vi "Acquire.vi"(8 "error in (no error)":errorcluster, 10 "Capacitive Readout Notifier":refnum<notifier>, 11 "Hardware Refs In":T1={"IP Address"="Simulator", "Handle"=0, "Refresh Time (ms)"=0.0}) -> (0 "error out":errorcluster, 3 "Hardware Refs Out":T1={"IP Address"="Simulator", "Handle"=0, "Refresh Time (ms)"=0.0})   [LabVIEW 2013, in "Capacitive.lvlib"]
uses:
  Capacitive.lvlib
  Hardware Configuration.ctl
  Capacitive Signal Cluster.ctl
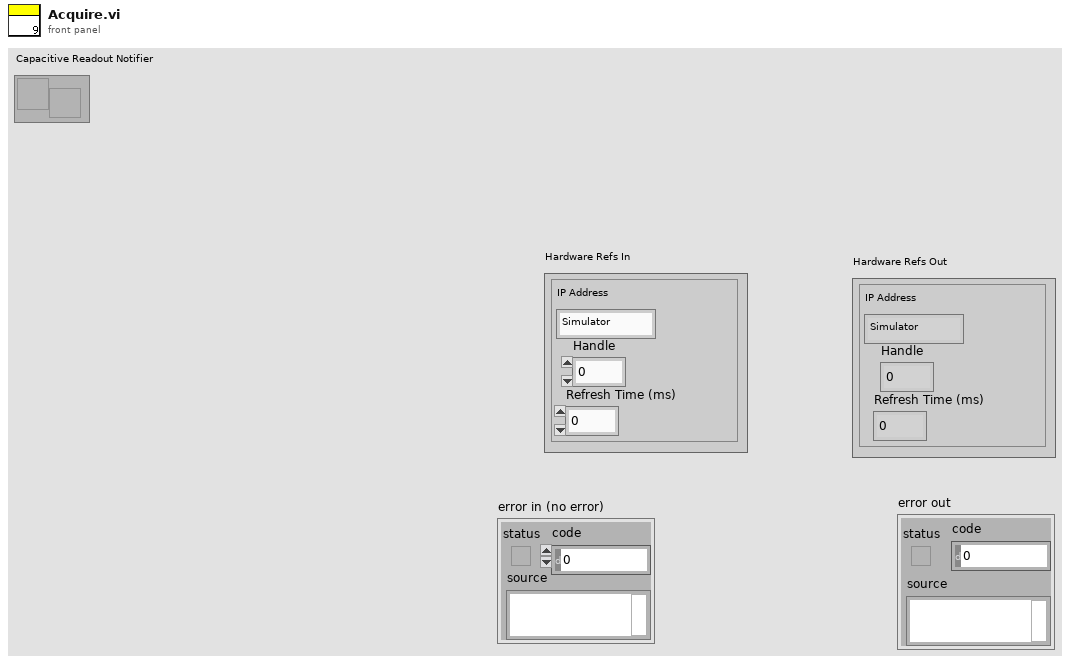
[diagram p1: front panel]
types:
  T1 = typedef "Capacitive.lvlib/Hardware Configuration.ctl" = cluster{"IP Address":string, "Handle":u32, "Refresh Time (ms)":dbl}
  T2 = typedef "Capacitive.lvlib/Capacitive Signal Cluster.ctl" = cluster{"Readout":sgl, "Time":i32, "Temperature":dbl}
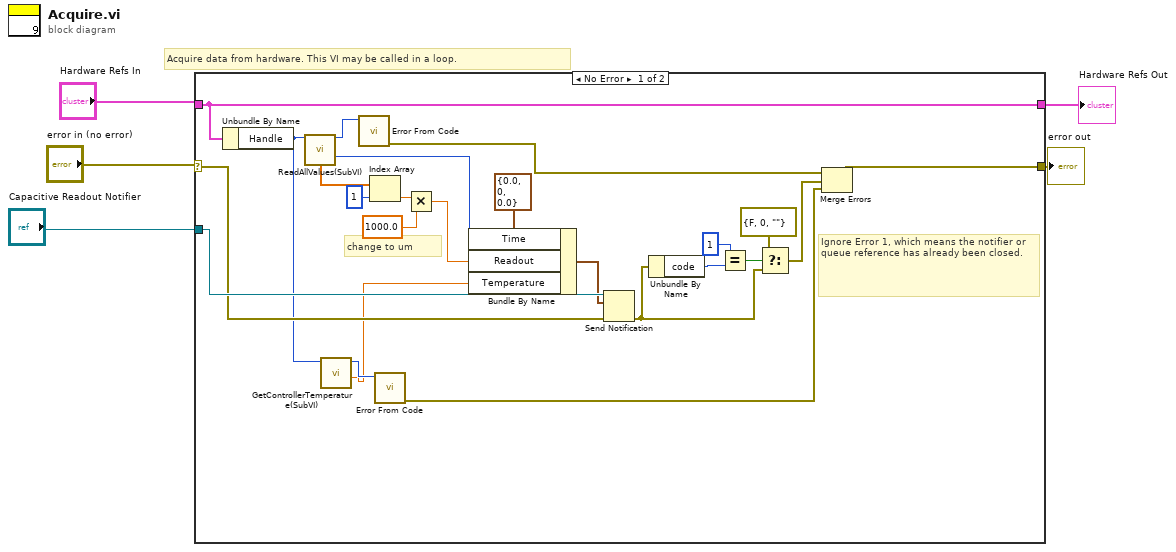
[diagram p0: block diagram]
diagram:
  # "Acquire data from hardware. This VI may be called in a loop."
  n1 = case shown="No Error" "error in (no error)" {
    selector: "error in (no error)" -> [w15 w30]
    tunnel: [w29 w30] -> w4
    tunnel: "Hardware Refs In" -> [w19 w31]
    tunnel: [w19 w31] -> w3
    tunnel: "Capacitive Readout Notifier" -> [w23 _]
    frame No Error {
      # "change to um"
      # "Ignore Error 1, which means the notifier or queue reference has already been closed."
      n2 = Unbundle By Name(w19) -> ("Handle"=w9:u32)
      n3 = call "ReadAllValues(SubVI).vi"("Handle in"=w9) -> ("Status"=w14:i32, "Timestamp"=w16:u64, "Displacement"=w18:dbl[])  [unwired: 8 in, 4 out]
      n4 = call "GetControllerTemperature(SubVI).vi"("Handle"=w9) -> ("Temperature"=w6:sgl, "Status"=w8:i32)  [unwired: 8 in, 1 out]
      n5 = call "Error From Code.vi"("ErrorCode"=w14) -> ("error out"=w13:errorcluster)  [unwired: 10 in]
      n6 = Index Array(array=w18, index=1) -> (element=w12:dbl)
      n7 = call "Error From Code.vi"("ErrorCode"=w8) -> ("error out"=w7:errorcluster)  [unwired: 10 in]
      n8 = Multiply(x=w12, y=1000.0) -> (x*y=w11:dbl)
      n9 = Bundle By Name(cluster=T2 {"Readout"=0.0, "Time"=0, "Temperature"=0.0} ("Capacitive Signal Cluster"), "Time"=w16, "Readout"=w11, "Temperature"=w6) -> (w21:T2)
      n10 = Send Notification(notification=w21, notifier=w23, error in (no error)=w15) -> (error out=w22:errorcluster)  [unwired: 1 out]
      n11 = Unbundle By Name(w22) -> ("code"=w28:i32)
      n12 = Equal?(x=1, y=w28) -> (x = y?=w26:bool)
      n13 = Select(t=errorcluster {"status"=FALSE, "code"=0, "source"=""} ("error constant"), s=w26, f=w22) -> (s? t:f=w25:errorcluster)
      n14 = Merge Errors(w13, w25, w7) -> (w29:errorcluster)
    }
    frame Error {
    }
  }
  "error out" <- w4
  "Hardware Refs Out" <- w3
